vi "Run-Time Menu - Toggle API Tester Enabled--helper.vi"(8 "error in (no error)":errorcluster, 10 "enabled":bool, 11 "Menu in":refnum<k9>) -> (0 "error out":errorcluster)   [LabVIEW 2022 SP3, in "UI Manager.lvlib"]
doc: "____\nHAMPEL SOFTWARE ENGINEERING v2.6.0 (2023-12-19 10:54)"
uses:
  UI Manager.lvlib
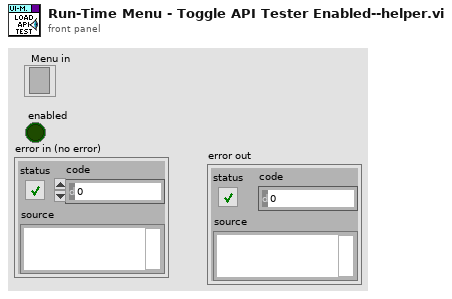
[diagram p1: front panel]
types:
  T1 = typedef "LVMenuShortCut.ctl" = cluster{"include Shift key?":bool, "include Ctrl key?":bool, "shortcut key":string}
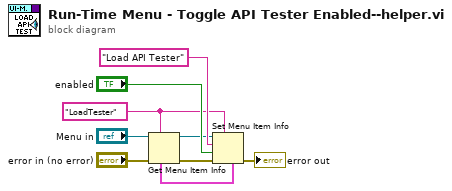
[diagram p0: block diagram]
diagram:
  w7 = "LoadTester" ("format string")
  n1 = Get Menu Item Info(7:w7, 8:"error in (no error)", 11:"Menu in") -> (0:w5:errorcluster, 3:w1:refnum<k9>, 6:w6:T1)  [unwired: 4 out]
  n2 = Set Menu Item Info(4:w6, 7:w7, 8:w5, 9:"enabled", 10:"Load API Tester" ("format string"), 11:w1) -> (0:→"error out":errorcluster)  [unwired: 1 in, 1 out]
